vi "ComPort.vi"(2 "stop bits (10: 1 bit)":u16(ring)=10 items=["1.0"=10, "1.5"=15, "2.0"=20], 5 "parity (0:none)":enum16{"None", "Odd", "Even", "Mark", "Space"}(ring), 6 "write buffer":string, 7 "ComAction":T1, 8 "error in (no error)":errorcluster, 9 "data bits (8)":u16=8 min=5 max=8 step=1, 10 "baud rate (9600)":u32=9600, 11 "VISA resource name":refnum<visa-resource-name>) -> (0 "error out":errorcluster, 3 "VISA resource name out":refnum<visa-resource-name>, 4 "read buffer":string)   [LabVIEW 2019]
uses:
  ComPortActionTypeDef.ctl
  <vilib>/Instr/_visa.llb/VISA Configure Serial Port (Instr).vi
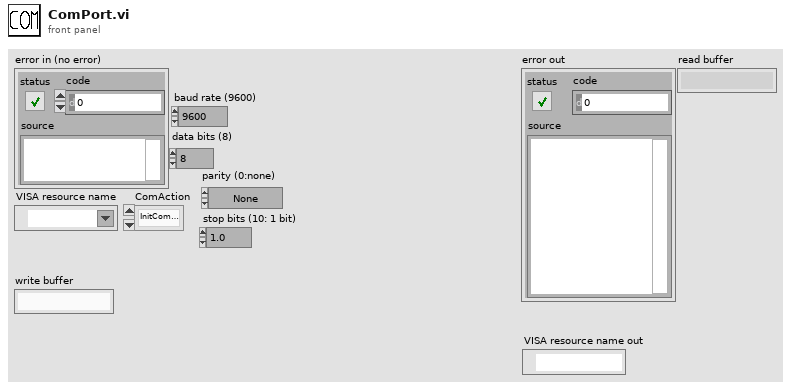
[diagram p1: front panel]
types:
  T1 = typedef "ComPortActionTypeDef.ctl" = enum16{"InitComPort", "ReadComPort", "WriteComePort", "CloseComPort"}
  T2 = enum16{"open", "replace", "create", "open or create", "replace or create", "replace or create with confirmation"}
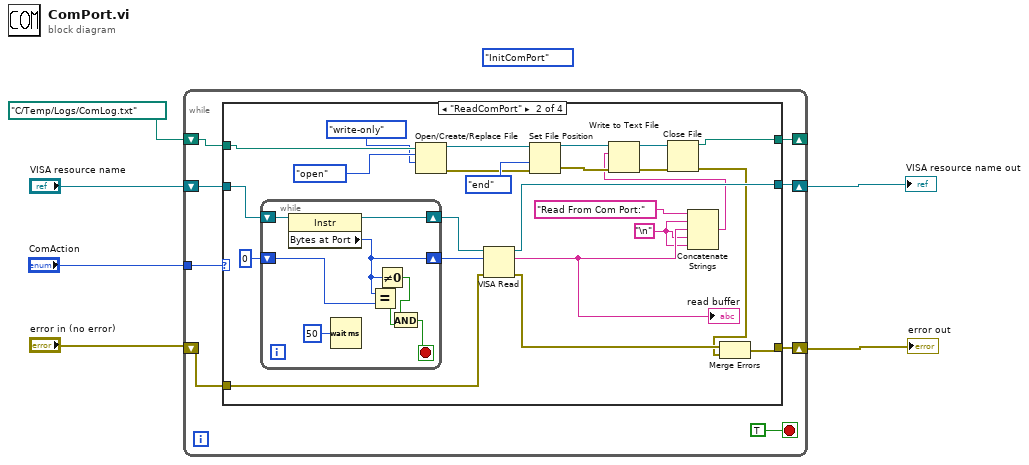
[diagram p0: block diagram]
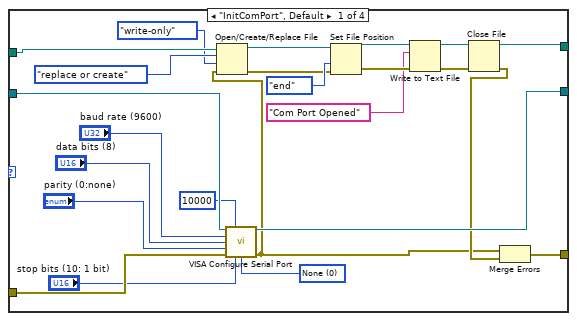
[diagram p2: hidden frame]
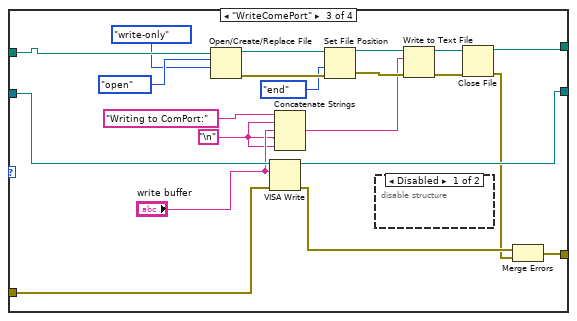
[diagram p3: hidden frame]
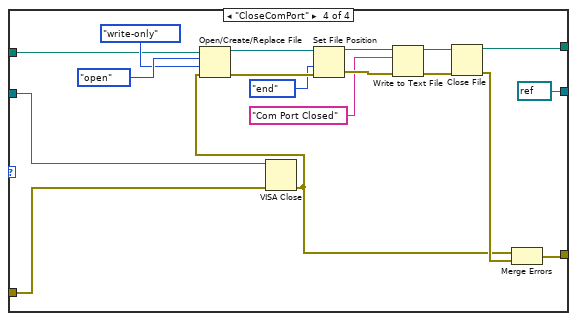
[diagram p5: hidden frame]
diagram:
  (unwired) ComPortActionTypeDef."InitComPort"
  n1 = while {
    tunnel: "ComAction" -> [w13]
    shift-right: [w11] -> w4
    shift-left: "error in (no error)" -> [w12]
    shift-right: [w9] -> w2
    shift-left: "VISA resource name" -> [w10]
    shift-right: [w8] -> _
    shift-left: path "C:/Temp/Logs/ComLog.txt" ("Path") -> [w7]
    stop <- TRUE stop-if-true
    n2 = case shown="\"ReadComPort\"" w13 {
      tunnel: w12 -> [w38 w60 w89 w108]
      tunnel: [w17 w41 w73 w94] -> w11
      tunnel: w10 -> [w37 w62 w91 w109]
      tunnel: [w32 w61 w90 refnum<visa-resource-name> refnum ("VISA resource name")] -> w9
      tunnel: [w25 w49 w81 w97] -> w8
      tunnel: w7 -> [w20 w53 w82 w96]
      frame "InitComPort", Default {
        w30 = u16 0 items=["None", "XON/XOFF", "RTS/CTS", "XON/XOFF & RTS/CTS", "DTR/DSR", "XON/XOFF & DTR/DSR"] ("flow control (0:none)")
        n3 = call-poly "VISA Configure Serial Port"("VISA resource name"=w37, "timeout (10sec)"=u32 10000, "baud rate (9600)"="baud rate (9600)", "data bits (8)"="data bits (8)", "parity (0:none)"="parity (0:none)", "error in (no error)"=w38, "stop bits (10: 1 bit)"="stop bits (10: 1 bit)", "flow control (0:none)"=w30) -> ("VISA resource name out"=w32:refnum<visa-resource-name>, "error out"=w15:errorcluster)  [unwired: 6 in]
        n4 = Open/Create/Replace File(file path (use dialog)=w20, error in=w15, operation (0:open)=T2."replace or create", access (0:read/write)=enum16{"read/write", "read-only", "write-only"}."write-only") -> (refnum out=w22:refnum<file>, error out=w21:errorcluster)  [unwired: 2 in, 1 out]
        n5 = Set File Position(refnum=w22, from (0:start)=enum16{"start", "end", "current"}."end", error in=w21) -> (refnum out=w29:refnum<file>, error out=w28:errorcluster)  [unwired: 1 in]
        n6 = Write to Text File(file (use dialog)=w29, text="Com Port Opened", error in=w28) -> (refnum out=w24:refnum<file>, error out=w23:errorcluster)  [unwired: 1 in, 1 out]
        n7 = Close File(refnum=w24, error in=w23) -> (path=w25:path, error out=w16:errorcluster)
        n8 = Merge Errors(w15, w16) -> (w17:errorcluster)
      }
      frame "ReadComPort" {
        w44 = "\n"
        n9 = while {
          shift-right: [w69] -> w59
          shift-left: w62 -> [w70]
          shift-right: [w68] -> w58
          shift-left: u32 0 ("Bytes at Port") -> [w67]
          stop <- w64 stop-if-true
          n10 = property class="Instr"(reference=w70) -> (reference out=w69:refnum<visa-resource-name>, "Bytes at Port"=w68:u32)  [unwired: 1 in, 1 out]
          n11 = Wait (ms)(milliseconds to wait=u32 50) -> ()  [unwired: 1 out]
          n12 = Equal?(x=w68, y=w67) -> (x = y?=w63:bool)
          n13 = Not Equal To 0?(x=w68) -> (x != 0?=w65:bool)
          n14 = And(x=w65, y=w63) -> (x .and. y?=w64:bool)
        }
        n15 = Open/Create/Replace File(file path (use dialog)=w53, operation (0:open)=T2."open", access (0:read/write)=enum16{"read/write", "read-only", "write-only"}."write-only") -> (refnum out=w52:refnum<file>, error out=w48:errorcluster)  [unwired: 3 in, 1 out]
        n16 = VISA Read(VISA resource name=w59, byte count=w58, error in (no error)=w60) -> (VISA resource name out=w61:refnum<visa-resource-name>, read buffer=w45:string, error out=w42:errorcluster)  [unwired: 1 out]
        "read buffer" <- w45
        n17 = Set File Position(refnum=w52, from (0:start)=enum16{"start", "end", "current"}."end", error in=w48) -> (refnum out=w57:refnum<file>, error out=w56:errorcluster)  [unwired: 1 in]
        n18 = Concatenate Strings("Read From Com Port:", w44, w45, w44, w44) -> (w43:string)
        n19 = Write to Text File(file (use dialog)=w57, text=w43, error in=w56) -> (refnum out=w50:refnum<file>, error out=w51:errorcluster)  [unwired: 1 in, 1 out]
        n20 = Close File(refnum=w50, error in=w51) -> (path=w49:path, error out=w40:errorcluster)
        n21 = Merge Errors(w42, w40) -> (w41:errorcluster)
      }
      frame "WriteComePort" {
        w76 = "\n"
        n22 = Open/Create/Replace File(file path (use dialog)=w82, operation (0:open)=T2."open", access (0:read/write)=enum16{"read/write", "read-only", "write-only"}."write-only") -> (refnum out=w85:refnum<file>, error out=w80:errorcluster)  [unwired: 3 in, 1 out]
        n23 = VISA Write(VISA resource name=w91, write buffer="write buffer", error in (no error)=w89) -> (VISA resource name out=w90:refnum<visa-resource-name>, error out=w72:errorcluster)  [unwired: 1 out]
        n24 = Concatenate Strings("Writing to ComPort:", w76, "write buffer", w76, w76) -> (w75:string)
        n25 = Set File Position(refnum=w85, from (0:start)=enum16{"start", "end", "current"}."end", error in=w80) -> (refnum out=w88:refnum<file>, error out=w87:errorcluster)  [unwired: 1 in]
        n26 = disable-structure shown="Disabled" {
          frame Disabled {
          }
          frame Enabled {
          }
        }
        n27 = Write to Text File(file (use dialog)=w88, text=w75, error in=w87) -> (refnum out=w83:refnum<file>, error out=w84:errorcluster)  [unwired: 1 in, 1 out]
        n28 = Close File(refnum=w83, error in=w84) -> (path=w81:path, error out=w71:errorcluster)
        n29 = Merge Errors(w72, w71) -> (w73:errorcluster)
      }
      frame "CloseComPort" {
        n30 = VISA Close(VISA resource name=w109, error in (no error)=w108) -> (error out=w92:errorcluster)
        n31 = Open/Create/Replace File(file path (use dialog)=w96, error in=w92, operation (0:open)=T2."open", access (0:read/write)=enum16{"read/write", "read-only", "write-only"}."write-only") -> (refnum out=w103:refnum<file>, error out=w100:errorcluster)  [unwired: 2 in, 1 out]
        n32 = Set File Position(refnum=w103, from (0:start)=enum16{"start", "end", "current"}."end", error in=w100) -> (refnum out=w106:refnum<file>, error out=w105:errorcluster)  [unwired: 1 in]
        n33 = Write to Text File(file (use dialog)=w106, text="Com Port Closed", error in=w105) -> (refnum out=w101:refnum<file>, error out=w102:errorcluster)  [unwired: 1 in, 1 out]
        n34 = Close File(refnum=w101, error in=w102) -> (path=w97:path, error out=w93:errorcluster)
        n35 = Merge Errors(w92, w93) -> (w94:errorcluster)
      }
    }
  }
  "error out" <- w4
  "VISA resource name out" <- w2
